vi "Init.vi"(8 "error in (no error)":errorcluster, 10 "Instrument String":variant, 11 "Lambda Gen Plus in":refnum<class "Lambda Gen Plus.lvclass">) -> (0 "error out":errorcluster, 2 "Found?":bool, 3 "Lambda Gen Plus out":refnum<class "Lambda Gen Plus.lvclass">)   [LabVIEW 2025, in "Power Supply.lvlib" / "Lambda Gen Plus.lvclass"]
uses:
  Lambda Gen Plus.lvclass
  Lambda Gen Plus.lvclass/Lambda Gen Plus.ctl
  Users/Public/Documents/Sandia National Labs/TSS Plugin/Abstract Engine.lvlibp/Instrument configuration/Instrument configuration.lvclass
  <instrlib>/TDK-Lambda G Series/TDK-Lambda G Series.lvlib
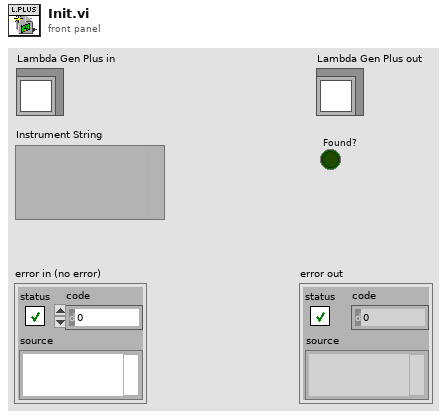
[diagram p1: front panel]
types:
  T1 = typedef "Abstract Engine.lvlibp/Instrument configuration.lvclass/Default Instrument.ctl" = cluster{"Type":string, "Address":string, "SW Alias":string, "Description":string, "Enabled":bool}
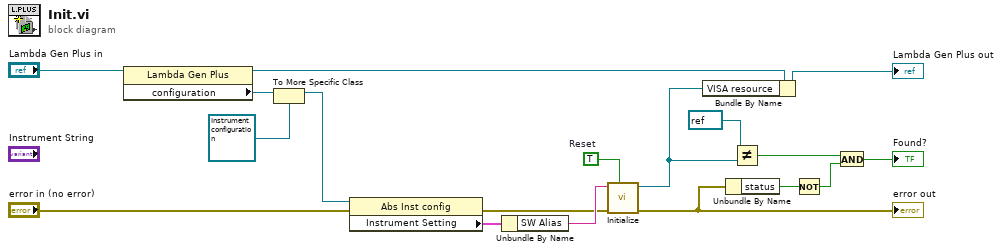
[diagram p0: block diagram]
diagram:
  w1 = TRUE  # Reset
  n1 = property class="Lambda Gen Plus"(reference="Lambda Gen Plus in") -> (reference out=w12:refnum<class "Lambda Gen Plus.lvclass">, "configuration"=w15:refnum<class "CEF_serializable configuration.lvclass">)  [unwired: 1 in, 1 out]
  n2 = To More Specific Class(target class=refnum<class "Instrument configuration.lvclass"> refnum ("Abstract PlugIn.lvlibp:Instrument configuration"), reference=w15) -> (specific class reference=w14:refnum<class "Instrument configuration.lvclass">)  [unwired: 1 in, 1 out]
  n3 = property class="Abs Inst config"(reference=w14, error in="error in (no error)") -> (error out=w9:errorcluster, "Instrument Setting"=w2:T1)  [unwired: 1 out]
  n4 = Unbundle By Name(w2) -> ("SW Alias"=w11:string)
  n5 = call <instrlib>:"Initialize.vi"("Reset (True)"=w1, "error in (no error)"=w9, "VISA resource name"=w11) -> ("error out"=w7:errorcluster, "VISA resource name out"=w17:refnum<visa-resource-name>)  [unwired: 7 in]
  "error out" <- w7
  n6 = Bundle By Name(cluster=w12, "VISA resource"=w17) -> (→"Lambda Gen Plus out":refnum<class "Lambda Gen Plus.lvclass">)
  n7 = Unbundle By Name(w7) -> ("status"=w6:bool)
  n8 = Not Equal?(x=refnum<visa-resource-name> refnum ("VISA resource name out"), y=w17) -> (x != y?=w5:bool)
  n9 = Not(x=w6) -> (.not. x?=w8:bool)
  n10 = And(x=w5, y=w8) -> (x .and. y?=→"Found?":bool)
